vi "Config Differential Frame.vi"(10 "subpanel to main command event":T1, 11 "main to subpanel command event reg":T2) -> ()   [LabVIEW 2017, in "NI_Robotics_Configure Steering Frame.lvlib" / "Differential Frame Subpanel.lvlib"]
uses:
  <vilib>/robotics/Dialog/Configure Steering Frame/Differential Frame Subpanel/Differential Frame Subpanel.lvlib
  <vilib>/robotics/Dialog/Configure Steering Frame/Main to Subpanel Command Event Reg.ctl
  <vilib>/robotics/Dialog/Configure Steering Frame/Main to Subpanel Command.ctl
  <vilib>/robotics/Steering/Steering Frame/NI_Robotics_Steering Frame.lvclass
  <vilib>/robotics/Dialog/Configure Steering Frame/Subpanel to Main Command Event.ctl
  <vilib>/robotics/Dialog/Configure Steering Frame/Subpanel to Main Command.ctl
  <vilib>/robotics/Dialog/Configure Steering Frame/Differential Frame Subpanel/FP Refs.ctl
  <vilib>/robotics/Steering/Differential Steering Frame/NI_Robotics_Differential Steering Frame.lvclass
  c:/Program Files (x86)/National Instruments/LabVIEW 2017/vi.lib/robotics/Steering/Steering Frame/NI_Robotics_Steering Frame.lvclass
  <vilib>/robotics/Dialog/Configure Steering Frame/Send Update Picture Command.vi
  <vilib>/robotics/Dialog/Configure Steering Frame/Generate Subpanel to Main Event.vi
  <vilib>/Utility/error.llb/Clear Errors.vi
  <vilib>/robotics/Steering/Steering Frame/Set All Gear Ratio.vi
  <vilib>/robotics/Steering/Steering Frame/Set All Wheel Radius.vi
  <vilib>/robotics/Dialog/Configure Steering Frame/NI_Robotics_Configure Steering Frame.lvlib
panel:
  in  "Wheel Separation":dbl
  in  "Gear Ratio":dbl
  in  "Wheel Radius":dbl
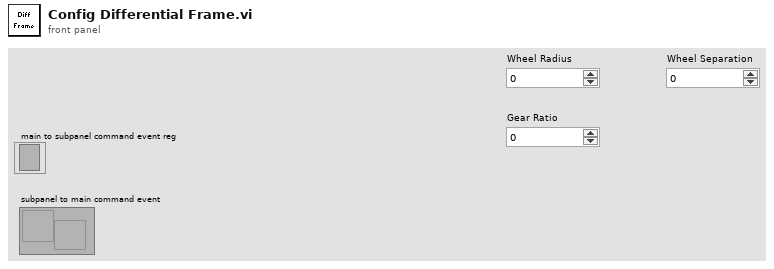
[diagram p1: front panel]
types:
  T1 = typedef "NI_Robotics_Configure Steering Frame.lvlib/Subpanel to Main Command Event.ctl" = refnum<user-event>
  T2 = typedef "NI_Robotics_Configure Steering Frame.lvlib/Main to Subpanel Command Event Reg.ctl" = refnum<event-registration>
  T3 = typedef "NI_Robotics_Configure Steering Frame.lvlib/Differential Frame Subpanel.lvlib/FP Refs.ctl" = cluster{"VI Refnum":refnum<vi>, "Wheel Radius":refnum<vi>, "Gear Ratio":refnum<vi>, "Wheel Separation":refnum<vi>}
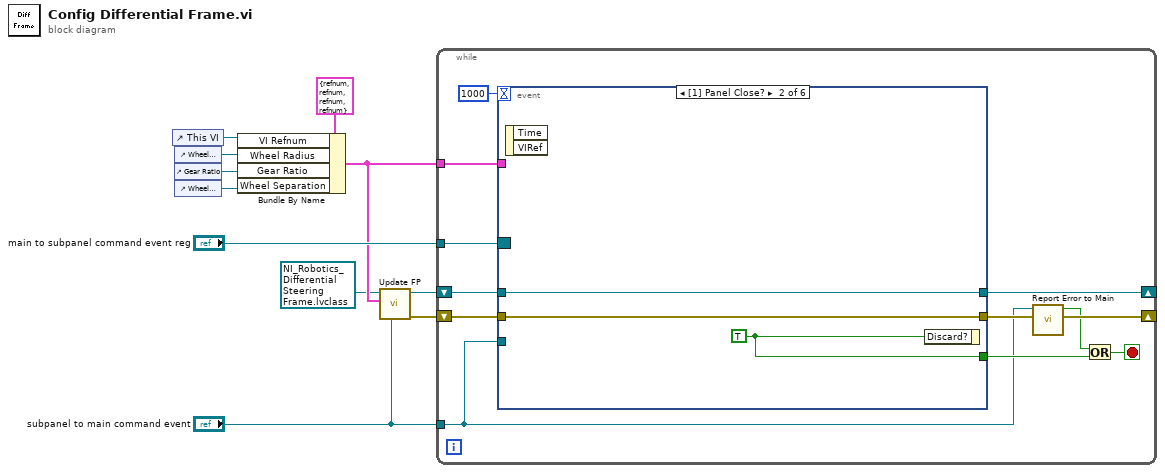
[diagram p0: block diagram]
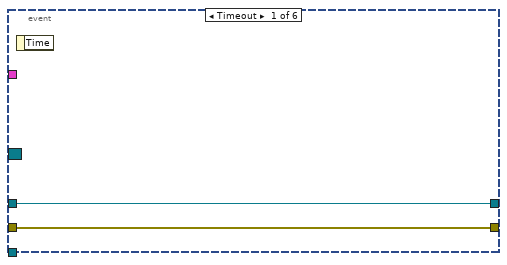
[diagram p2: hidden frame]
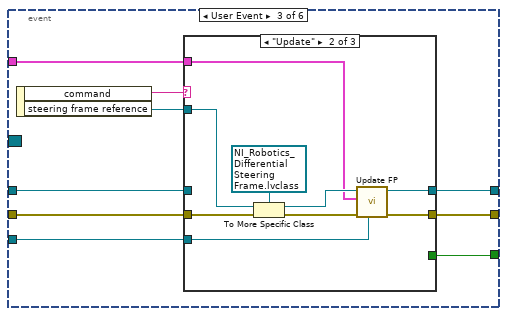
[diagram p3: hidden frame]
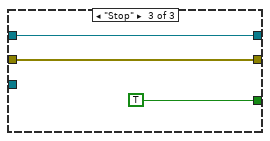
[diagram p5: hidden frame]
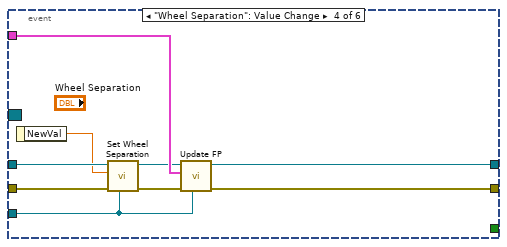
[diagram p6: hidden frame]
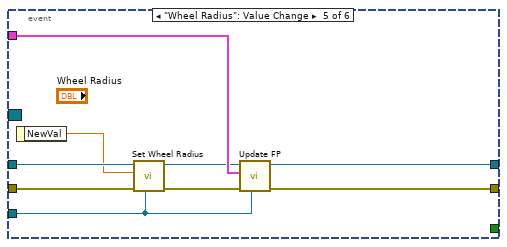
[diagram p7: hidden frame]
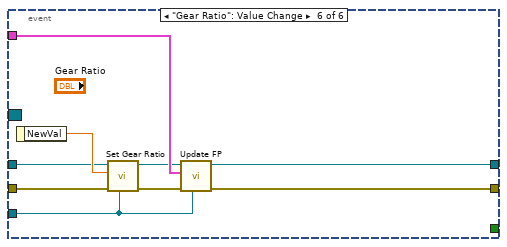
[diagram p8: hidden frame]
diagram:
  n1 = control-ref of="This VI"() -> (w8:refnum<vi>)
  n2 = control-ref of="Wheel Radius"() -> (w7:refnum<vi>)
  n3 = control-ref of="Gear Ratio"() -> (w6:refnum<vi>)
  n4 = control-ref of="Wheel Separation"() -> (w5:refnum<vi>)
  n5 = Bundle By Name(cluster=T3 {"VI Refnum"=refnum, "Wheel Radius"=refnum, "Gear Ratio"=refnum, "Wheel Separation"=refnum} ("fp refs"), "VI Refnum"=w8, "Wheel Radius"=w7, "Gear Ratio"=w6, "Wheel Separation"=w5) -> (w3:T3)
  n6 = call <vilib>:"Update FP.vi"("subpanel to main command event"="subpanel to main command event", "fp refs"=w3, "steering frame ref in"=refnum<data-value> refnum) -> ("error out"=w1:errorcluster, "steering frame ref out"=w4:refnum<data-value>)  [unwired: 7 in]
  n7 = while {
    shift-right: [w15] -> _
    shift-left: w1 -> [w23]
    tunnel: "main to subpanel command event reg" -> [w21]
    shift-right: [w20] -> _
    shift-left: w4 -> [w19]
    tunnel: "subpanel to main command event" -> [w12]
    tunnel: w3 -> [w16]
    stop <- w17 stop-if-true
    n8 = event shown="[1] Panel Close?" {
      selector: w21 -> [_ _ _ _ _ _]
      dyn-events: _ -> [_ _ _ _ _ _]
      timeout: 1000 -> [_ _ _ _ _ _]
      tunnel: w23 -> [w25 w28 w35 w59 w64 w72]
      tunnel: [w25 w28 w34 w53 w68 w76] -> w14
      tunnel: [w24 w27 w33 w55 w69 w77] -> w20
      tunnel: w19 -> [w24 w27 w32 w60 w66 w73]
      tunnel: [_ w26 w31 _ _ _] -> w18
      tunnel: w12 -> [_ _ w30 w52 w61 w70]
      tunnel: w16 -> [_ _ w29 w57 w67 w78]
      event Timeout {
        n9 = event-data() -> ()  [unwired: 1 in, 1 out]
      }
      event Panel Close? {
        w26 = TRUE ("Discard?")
        n10 = event-data() -> ()  [unwired: 1 in, 2 out]
        n11 = event-data("Discard?"=w26) -> ()  [unwired: 1 in, 1 out]
      }
      event User Event {
        n12 = event-data() -> ("command"=w37:string, "steering frame reference"=w36:refnum<data-value>)  [unwired: 1 in]
        n13 = case shown="\"Update\"" w37 {
          tunnel: w36 -> [_ w47 _]
          tunnel: w35 -> [w39 w46 w50]
          tunnel: [w39 w42 w50] -> w34
          tunnel: [w38 w44 w51] -> w33
          tunnel: w32 -> [w38 _ w51]
          tunnel: [_ _ TRUE] -> w31
          tunnel: w30 -> [_ w40 _]
          tunnel: w29 -> [_ w41 _]
          frame Default {
          }
          frame "Update" {
            n14 = To More Specific Class(target class=refnum<data-value> refnum ("data value reference"), reference=w47, error in=w46) -> (specific class reference=w45:refnum<data-value>, error out=w43:errorcluster)
            n15 = call <vilib>:"Update FP.vi"("subpanel to main command event"=w40, "error in (no error)"=w43, "fp refs"=w41, "steering frame ref in"=w45) -> ("error out"=w42:errorcluster, "steering frame ref out"=w44:refnum<data-value>)  [unwired: 6 in]
          }
          frame "Stop" {
          }
        }
      }
      event "Wheel Separation": Value Change {
        n16 = event-data() -> ("NewVal"=w58:dbl)  [unwired: 1 in]
        n17 = call <vilib>:"Set Wheel Separation.vi"("subpanel to main command event"=w52, "error in (no error)"=w59, "wheel separation"=w58, "steering frame ref in"=w60) -> ("error out"=w54:errorcluster, "steering frame ref out"=w56:refnum<data-value>)  [unwired: 6 in]
        n18 = call <vilib>:"Update FP.vi"("subpanel to main command event"=w52, "error in (no error)"=w54, "fp refs"=w57, "steering frame ref in"=w56) -> ("error out"=w53:errorcluster, "steering frame ref out"=w55:refnum<data-value>)  [unwired: 6 in]
      }
      event "Wheel Radius": Value Change {
        n19 = event-data() -> ("NewVal"=w62:dbl)  [unwired: 1 in]
        n20 = call <vilib>:"Set Wheel Radius.vi"("subpanel to main command event"=w61, "error in (no error)"=w64, "wheel radius"=w62, "steering frame ref in"=w66) -> ("error out"=w63:errorcluster, "steering frame ref out"=w65:refnum<data-value>)  [unwired: 6 in]
        n21 = call <vilib>:"Update FP.vi"("subpanel to main command event"=w61, "error in (no error)"=w63, "fp refs"=w67, "steering frame ref in"=w65) -> ("error out"=w68:errorcluster, "steering frame ref out"=w69:refnum<data-value>)  [unwired: 6 in]
      }
      event "Gear Ratio": Value Change {
        n22 = event-data() -> ("NewVal"=w75:dbl)  [unwired: 1 in]
        n23 = call <vilib>:"Set Gear Ratio.vi"("subpanel to main command event"=w70, "error in (no error)"=w72, "gear ratio"=w75, "steering frame ref in"=w73) -> ("error out"=w71:errorcluster, "steering frame ref out"=w74:refnum<data-value>)  [unwired: 6 in]
        n24 = call <vilib>:"Update FP.vi"("subpanel to main command event"=w70, "error in (no error)"=w71, "fp refs"=w78, "steering frame ref in"=w74) -> ("error out"=w76:errorcluster, "steering frame ref out"=w77:refnum<data-value>)  [unwired: 6 in]
      }
    }
    n25 = call <vilib>:"Report Error to Main.vi"("error in (no error)"=w14, "subpanel to main command event"=w12) -> ("error out"=w15:errorcluster, "reported error?"=w13:bool)  [unwired: 8 in]
    n26 = Or(x=w13, y=w18) -> (x .or. y?=w17:bool)
  }
